vi "test-faketoggle.vi"() -> ()   [LabVIEW 2016]
uses:
  C:/Users/sciollalab/Documents/Brandeis-BNL/LabVIEW_Codes/BNL_ThermomechanicalStave/AerotechLibraries/Bin/Aerotech.A3200.dll
  AerotechLibraries/Bin/Aerotech.A3200.dll
panel:
  in  "error in (no error)":errorcluster
  in  "Axis Speeds":T1={"X [mm/s]"=10.0, "Y [mm/s]"=10.0, "Z [mm/s]"=10.0}
  out "Moving":bool
  in  "Program Errors":errorcluster
  out "XYZ Stage Control":refnum<k24>
  out "Stave origin":T2
  in  "XYZ Stage Frame: Coordinates for calibration":T3={"Stave origin"={"X [mm]"=-706.0, "Y [mm]"=140.5, "Z [mm]"=-13.5}, "Autofocus"={"X [mm]"=-686.0, "Y [mm]"=130.0, "Z [mm]"=-18.0}, "Calib Pattern"={"X [mm]"=-566.0, "Y [mm]"=39.26, "Z [mm]"=-22.0}}
  out "Current stage position [mm]":cluster{"X":dbl, "Y":dbl, "Z":dbl}
  in  "Update jog increment":bool
  in  "Jog step size":T2={"X [mm]"=0.1, "Y [mm]"=0.1, "Z [mm]"=0.1}
  in  "Backward":bool
  in  "Reset position":bool
  in  "Left":bool
  in  "Right":bool
  in  "Confirm position":bool
  in  "Forward":bool
  out "element":string
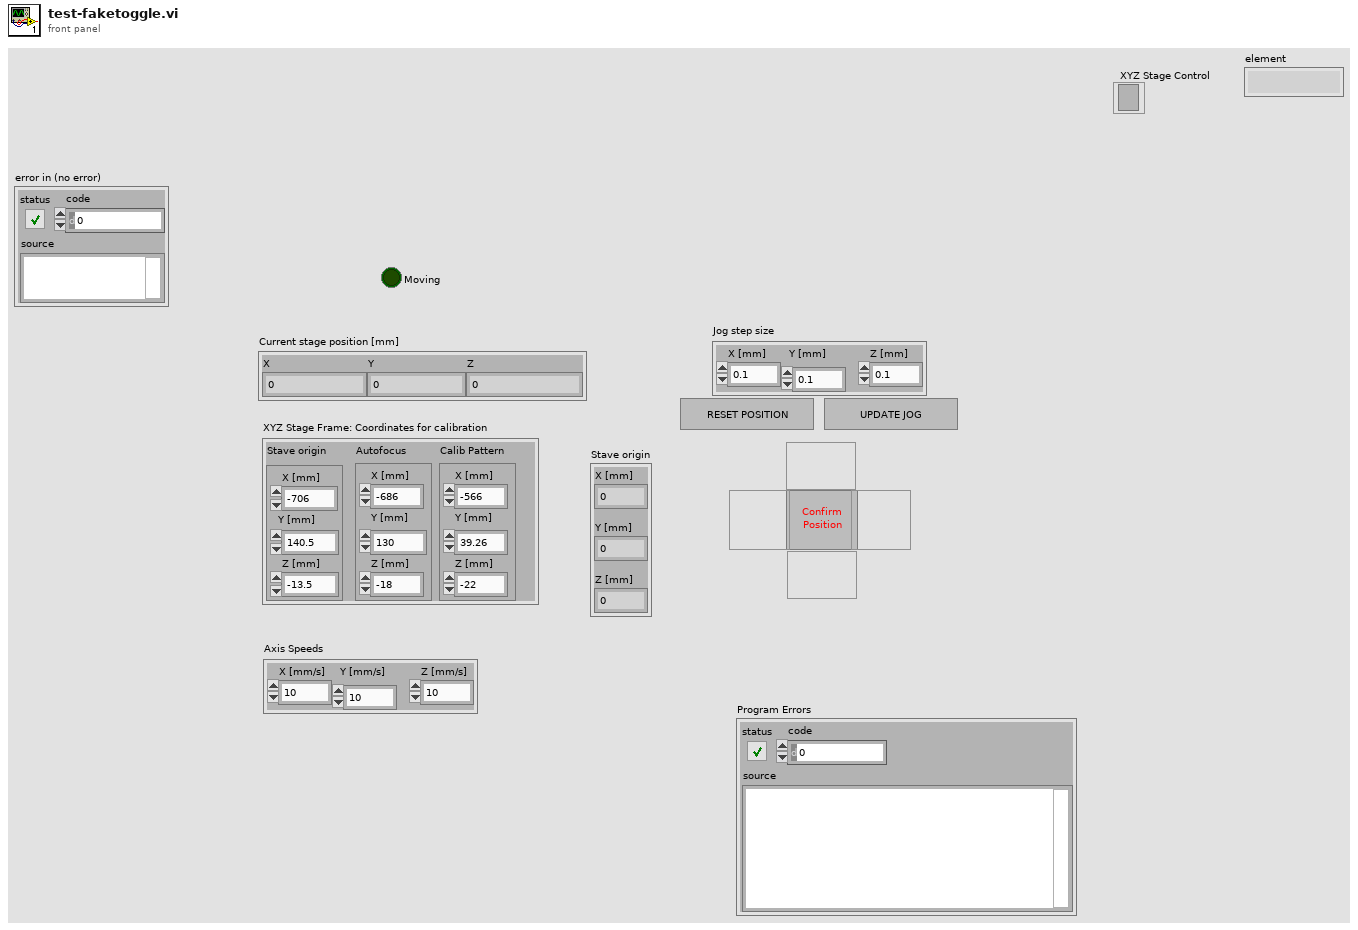
[diagram p1: front panel]
types:
  T1 = cluster{"X [mm/s]":dbl, "Y [mm/s]":dbl, "Z [mm/s]":dbl}
  T2 = cluster{"X [mm]":dbl, "Y [mm]":dbl, "Z [mm]":dbl}
  T3 = cluster{"Stave origin":cluster{"X [mm]":dbl, "Y [mm]":dbl, "Z [mm]":dbl}, "Autofocus":cluster{"X [mm]":dbl, "Y [mm]":dbl, "Z [mm]":dbl}, "Calib Pattern":cluster{"X [mm]":dbl, "Y [mm]":dbl, "Z [mm]":dbl}}
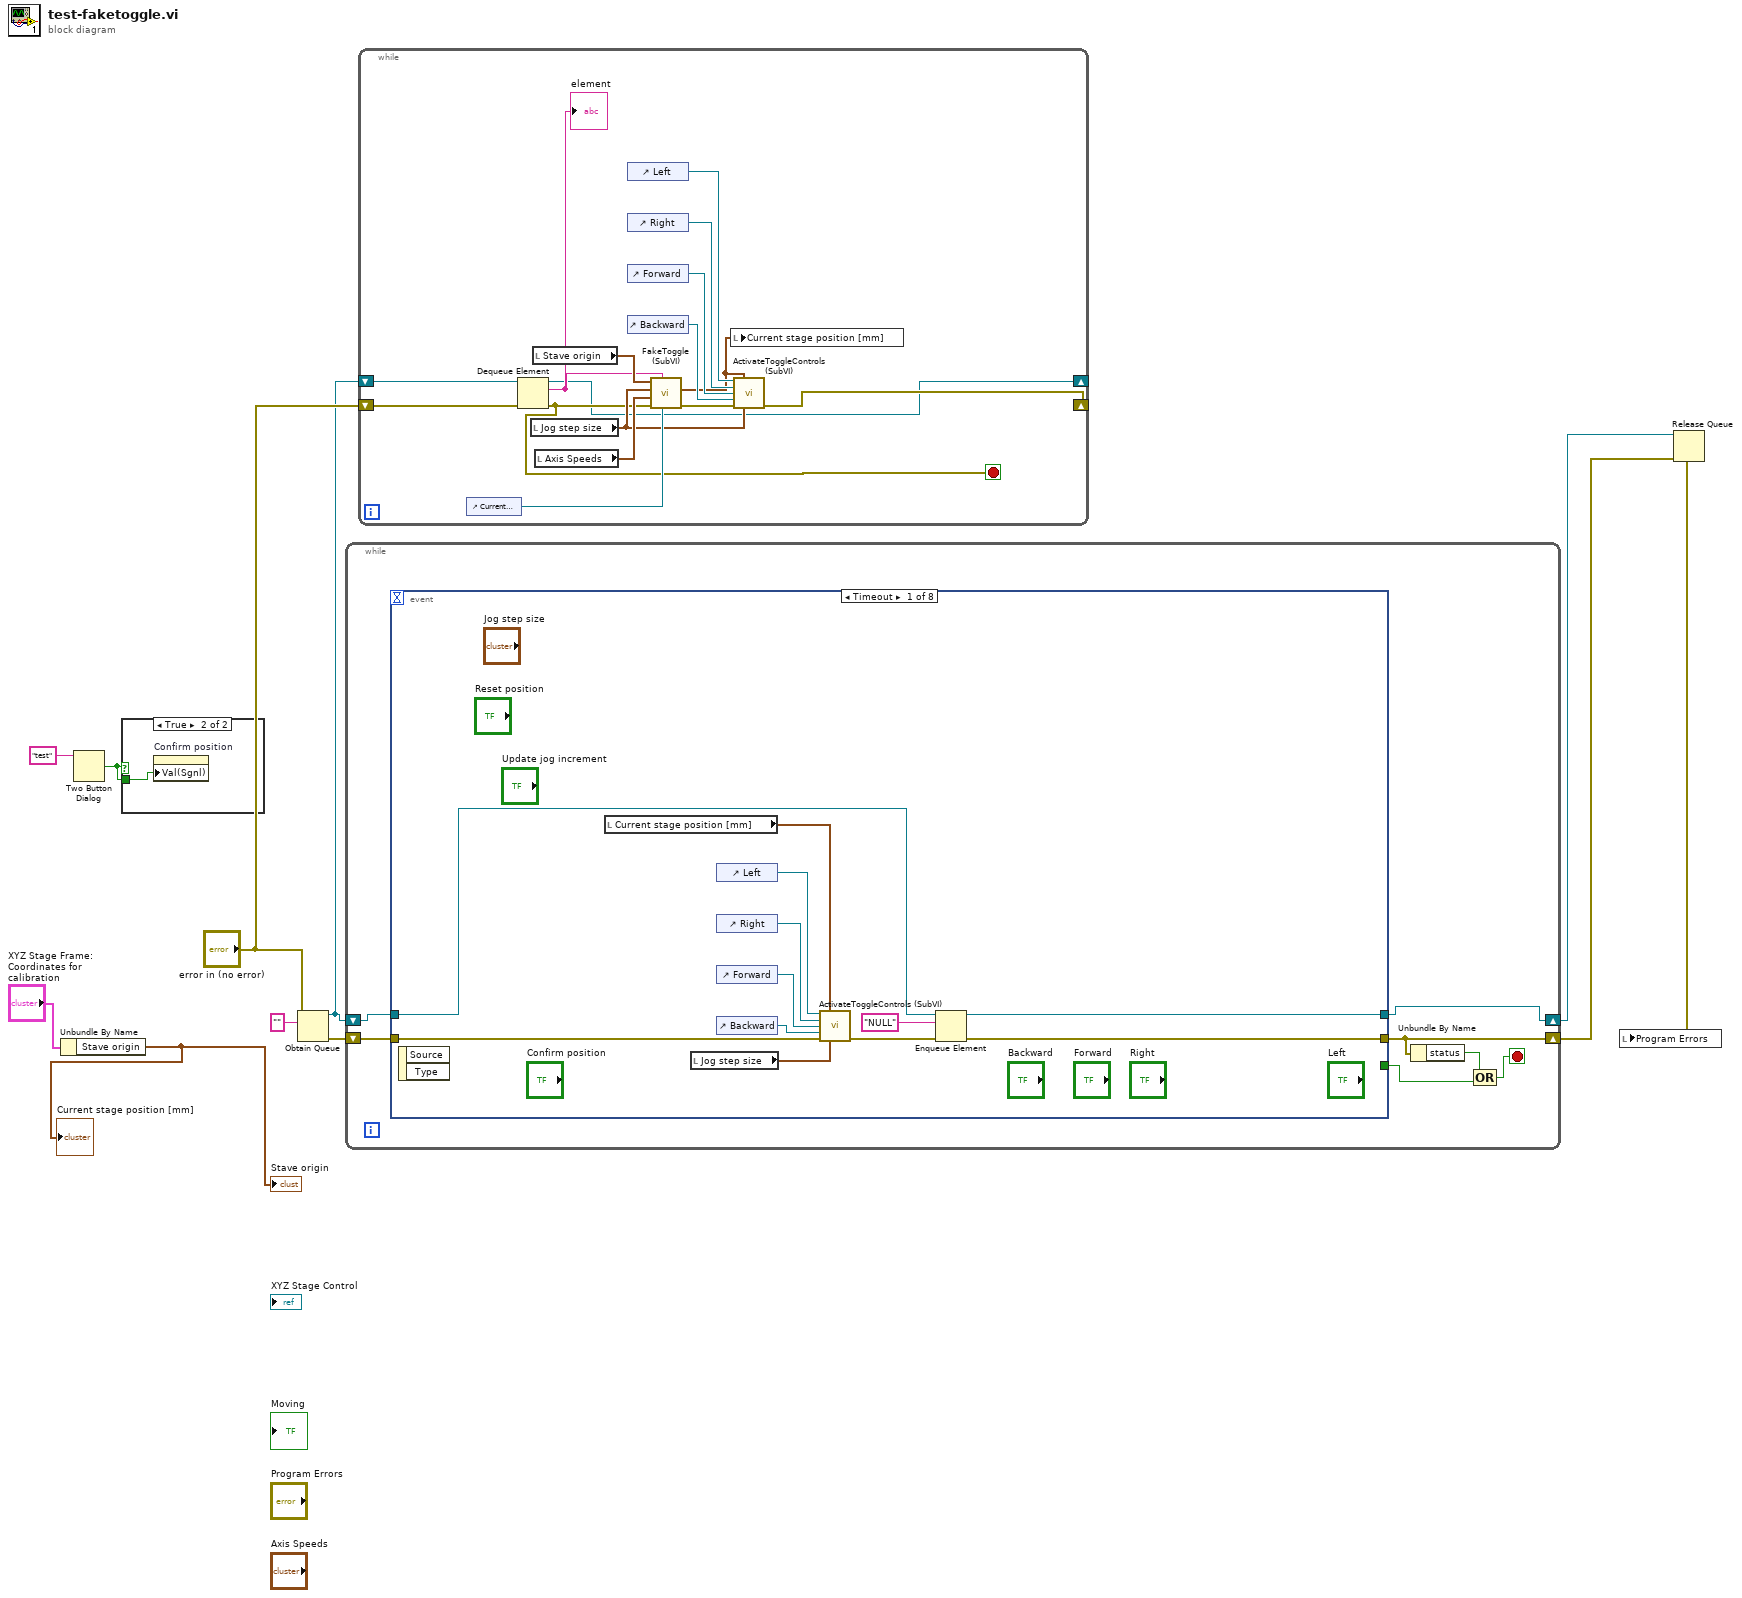
[diagram p0: block diagram]
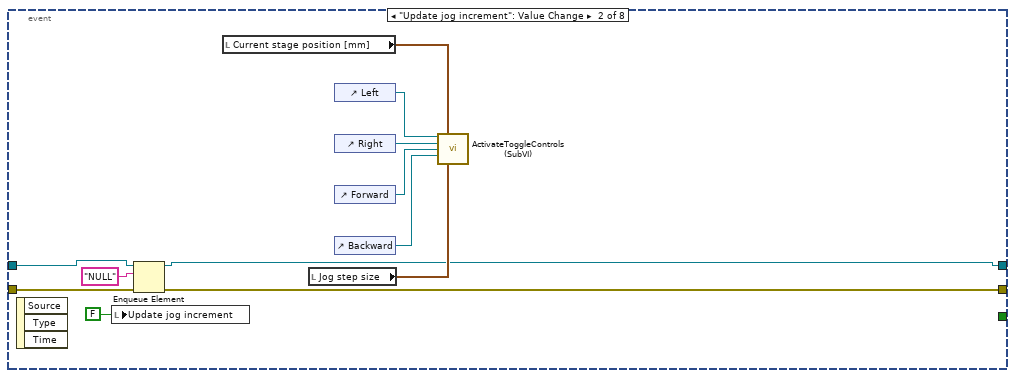
[diagram p3: hidden frame]
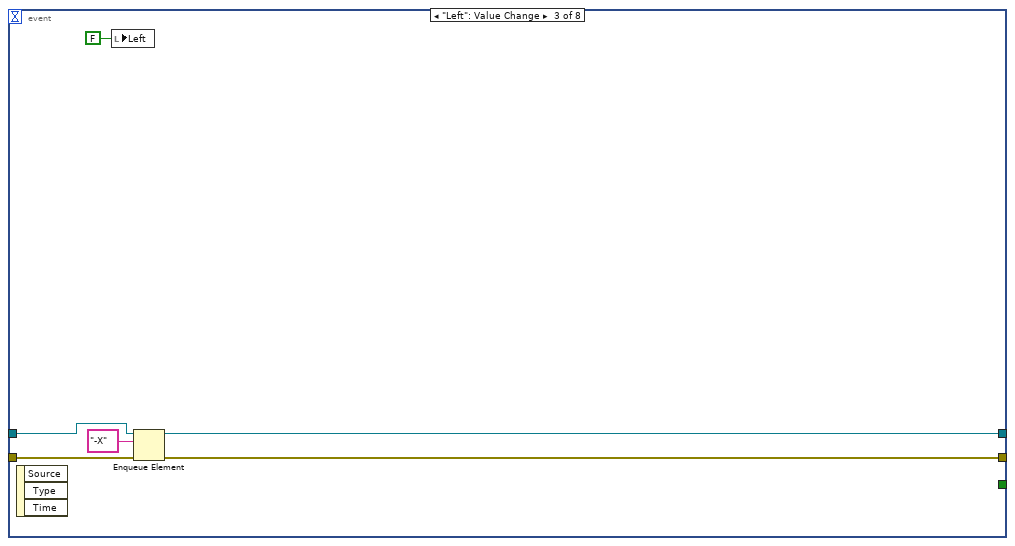
[diagram p4: hidden frame]
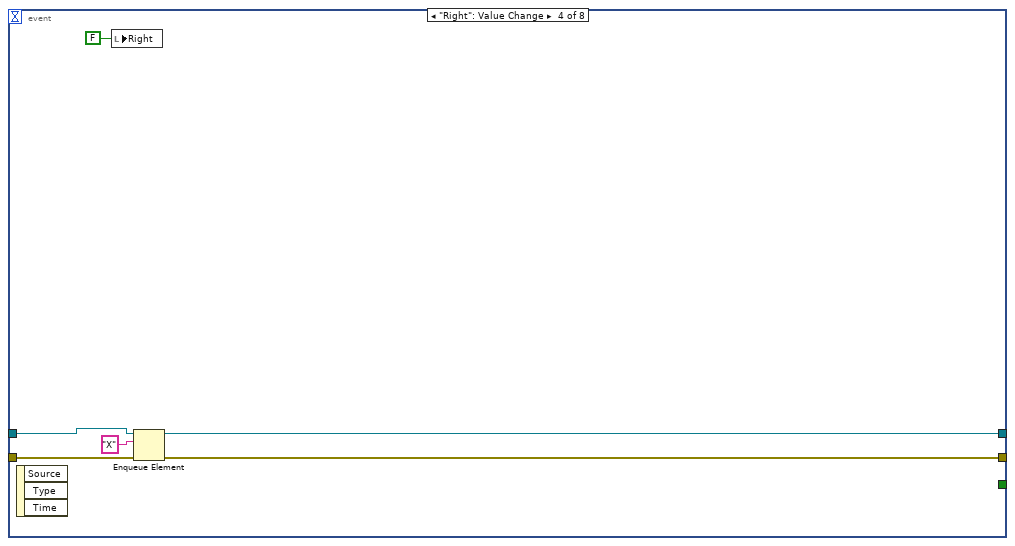
[diagram p5: hidden frame]
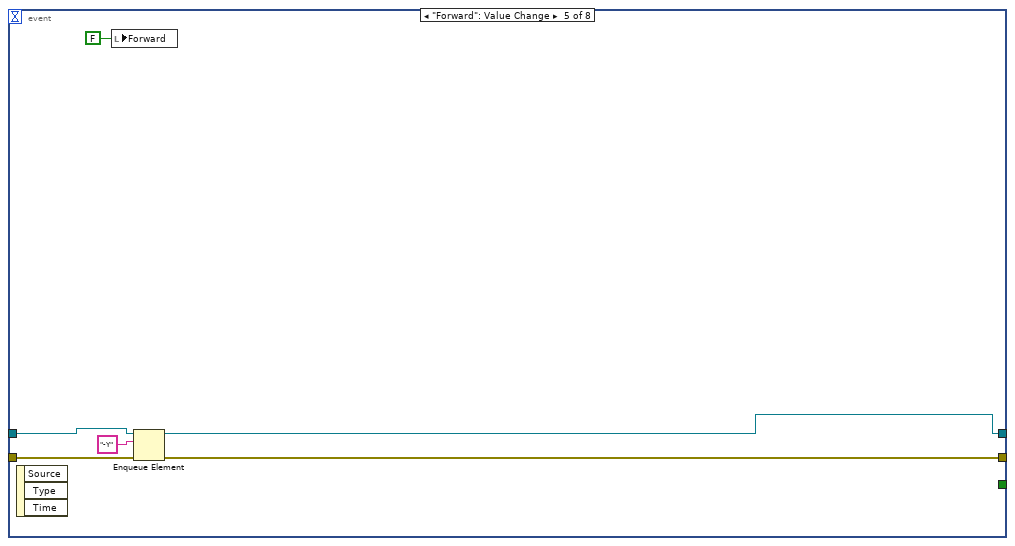
[diagram p6: hidden frame]
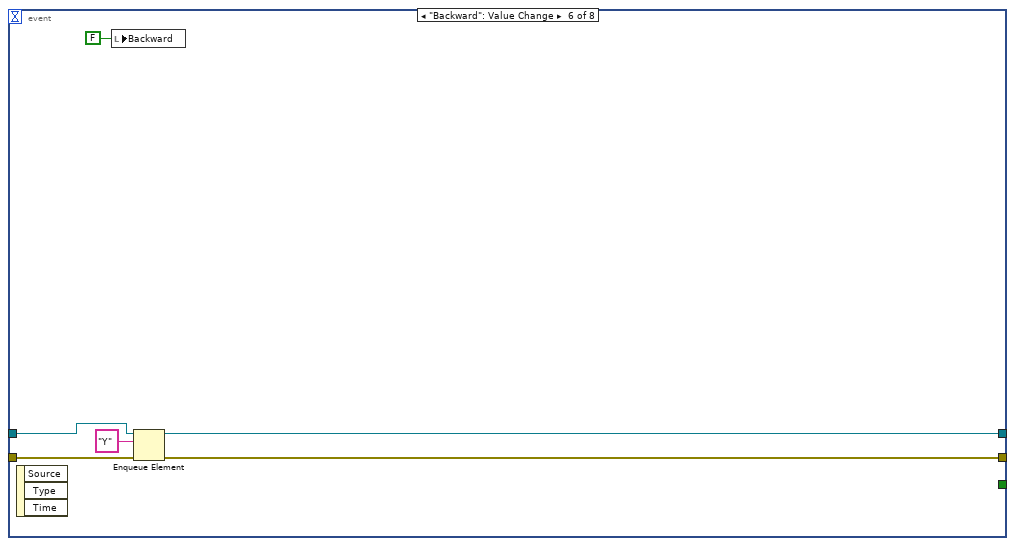
[diagram p7: hidden frame]
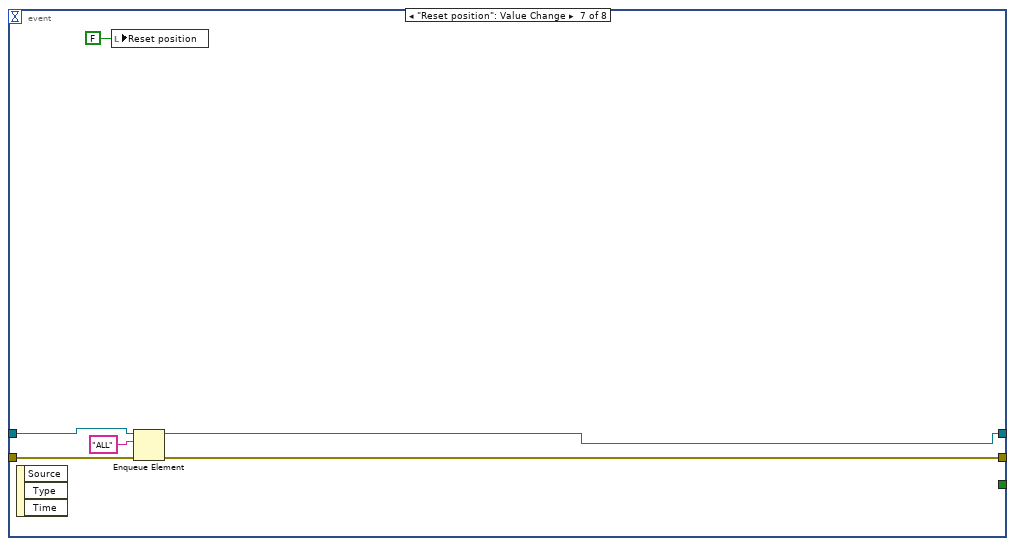
[diagram p8: hidden frame]
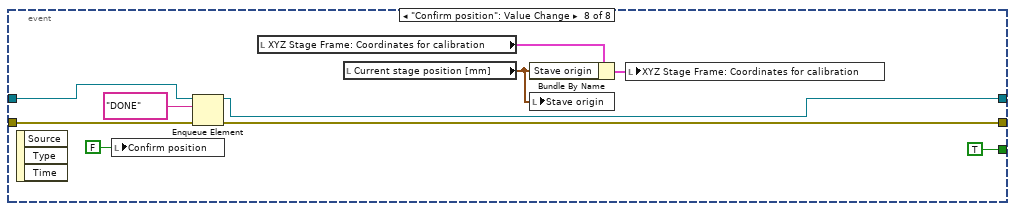
[diagram p9: hidden frame]
diagram:
  n1 = Unbundle By Name("XYZ Stage Frame: Coordinates for calibration") -> ("Stave origin"=→"Current stage position [mm]" →"Stave origin":T2)
  n2 = Two Button Dialog(message="test") -> (T button?=w1:bool)  [unwired: 2 in]
  n3 = case shown="True" w1 {
    tunnel: w1 -> [_ w12]
    frame False {
    }
    frame True {
      n4 = property on="Confirm position" class="Bool (strict)"("Val(Sgnl)"=w12) -> ()  [unwired: 2 in, 2 out]
    }
  }
  n5 = Obtain Queue(element data type="", error in (no error)="error in (no error)") -> (queue out=w5:refnum<queue>, error out=w11:errorcluster)  [unwired: 3 in, 1 out]
  n6 = while {
    shift-right: [w18] -> w3
    shift-left: w11 -> [w19]
    shift-right: [w13] -> w4
    shift-left: w5 -> [w14]
    stop <- w16 stop-if-true
    n7 = event shown="[0] Timeout" {
      selector: _ -> [_ _ _ _ _ _ _ _]
      dyn-events: _ -> [_ _ _ _ _ _ _ _]
      timeout: _ -> [_ _ _ _ _ _ _ _]
      tunnel: w14 -> [w24 w35 w47 w52 w60 w65 w72 w78]
      tunnel: w19 -> [w21 w34 w46 w54 w58 w64 w70 w75]
      tunnel: [w23 w33 w45 w53 w57 w63 w69 w76] -> w18
      tunnel: [_ _ _ _ _ _ _ TRUE] -> w15
      tunnel: [w20 w32 w44 w50 w56 w62 w68 w74] -> w13
      event Timeout {
        n8 = event-data() -> ()  [unwired: 1 in, 2 out]
        n9 = local read "Current stage position [mm]"() -> (w30:cluster{"X":dbl, "Y":dbl, "Z":dbl})
        n10 = local read "Jog step size"() -> (w31:T2)
        n11 = control-ref of="Left"() -> (w26:refnum<vi>)
        n12 = control-ref of="Right"() -> (w27:refnum<vi>)
        n13 = control-ref of="Forward"() -> (w28:refnum<vi>)
        n14 = control-ref of="Backward"() -> (w29:refnum<vi>)
        n15 = call "ActivateToggleControls (SubVI).vi"("Left refnum"=w26, "Current stage position [mm]"=w30, "Right refnum"=w27, "Forward refnum"=w28, "Backward refnum"=w29, "error in (no error)"=w21, "Jog step size"=w31) -> ("error out"=w22:errorcluster)  [unwired: 8 in]
        n16 = Enqueue Element(queue=w24, element="NULL", error in (no error)=w22) -> (queue out=w20:refnum<queue>, error out=w23:errorcluster)  [unwired: 1 in, 1 out]
      }
      event "Update jog increment": Value Change {
        n17 = event-data() -> ()  [unwired: 1 in, 3 out]
        n18 = local write "Update jog increment"(FALSE ("Update jog increment")) -> ()
        n19 = Enqueue Element(queue=w35, element="NULL", error in (no error)=w34) -> (queue out=w32:refnum<queue>, error out=w33:errorcluster)  [unwired: 1 in, 1 out]
        n20 = local read "Current stage position [mm]"() -> (w38:cluster{"X":dbl, "Y":dbl, "Z":dbl})
        n21 = local read "Jog step size"() -> (w39:T2)
        n22 = control-ref of="Left"() -> (w40:refnum<vi>)
        n23 = control-ref of="Right"() -> (w41:refnum<vi>)
        n24 = control-ref of="Forward"() -> (w42:refnum<vi>)
        n25 = control-ref of="Backward"() -> (w43:refnum<vi>)
        n26 = call "ActivateToggleControls (SubVI).vi"("Left refnum"=w40, "Current stage position [mm]"=w38, "Right refnum"=w41, "Forward refnum"=w42, "Backward refnum"=w43, "Jog step size"=w39) -> ()  [unwired: 9 in, 1 out]
      }
      event "Left": Value Change {
        n27 = event-data() -> ()  [unwired: 1 in, 3 out]
        n28 = local write "Left"(FALSE ("Left")) -> ()
        n29 = Enqueue Element(queue=w47, element="-X", error in (no error)=w46) -> (queue out=w44:refnum<queue>, error out=w45:errorcluster)  [unwired: 1 in, 1 out]
      }
      event "Right": Value Change {
        n30 = event-data() -> ()  [unwired: 1 in, 3 out]
        n31 = local write "Right"(FALSE ("Left")) -> ()
        n32 = Enqueue Element(queue=w52, element="X", error in (no error)=w54) -> (queue out=w50:refnum<queue>, error out=w53:errorcluster)  [unwired: 1 in, 1 out]
      }
      event "Forward": Value Change {
        n33 = event-data() -> ()  [unwired: 1 in, 3 out]
        n34 = local write "Forward"(FALSE ("Left")) -> ()
        n35 = Enqueue Element(queue=w60, element="-Y", error in (no error)=w58) -> (queue out=w56:refnum<queue>, error out=w57:errorcluster)  [unwired: 1 in, 1 out]
      }
      event "Backward": Value Change {
        n36 = event-data() -> ()  [unwired: 1 in, 3 out]
        n37 = local write "Backward"(FALSE ("Left")) -> ()
        n38 = Enqueue Element(queue=w65, element="Y", error in (no error)=w64) -> (queue out=w62:refnum<queue>, error out=w63:errorcluster)  [unwired: 1 in, 1 out]
      }
      event "Reset position": Value Change {
        n39 = event-data() -> ()  [unwired: 1 in, 3 out]
        n40 = local write "Reset position"(FALSE ("Reset position")) -> ()
        n41 = Enqueue Element(queue=w72, element="ALL", error in (no error)=w70) -> (queue out=w68:refnum<queue>, error out=w69:errorcluster)  [unwired: 1 in, 1 out]
      }
      event "Confirm position": Value Change {
        n42 = event-data() -> ()  [unwired: 1 in, 3 out]
        n43 = local write "Confirm position"(FALSE ("Confirm position")) -> ()
        n44 = Enqueue Element(queue=w78, element="DONE", error in (no error)=w75) -> (queue out=w74:refnum<queue>, error out=w76:errorcluster)  [unwired: 1 in, 1 out]
        n45 = local read "XYZ Stage Frame: Coordinates for calibration"() -> (w81:T3)
        n46 = local read "Current stage position [mm]"() -> (w80:cluster{"X":dbl, "Y":dbl, "Z":dbl})
        n47 = Bundle By Name(cluster=w81, "Stave origin"=w80) -> (w82:T3)
        n48 = local write "Stave origin"(w80) -> ()
        n49 = local write "XYZ Stage Frame: Coordinates for calibration"(w82) -> ()
      }
    }
    n50 = Unbundle By Name(w18) -> ("status"=w17:bool)
    n51 = Compound Arithmetic op=OR(w17, w15) -> (w16:bool)
  }
  n52 = while {
    shift-right: [w85] -> _
    shift-left: "error in (no error)" -> [w87]
    shift-right: [w84] -> _
    shift-left: w5 -> [w99]
    stop <- w86 stop-if-true
    n53 = control-ref of="Current stage position [mm]"() -> (w96:refnum<vi>)
    n54 = Dequeue Element(queue=w99, error in (no error)=w87) -> (queue out=w84:refnum<queue>, element=w95:string, error out=w86:errorcluster)  [unwired: 1 in, 1 out]
    "element" <- w95
    n55 = local read "Jog step size"() -> (w89:T2)
    n56 = local read "Stave origin"() -> (w98:T2)
    n57 = local read "Axis Speeds"() -> (w97:T1)
    n58 = control-ref of="Left"() -> (w94:refnum<vi>)
    n59 = control-ref of="Right"() -> (w93:refnum<vi>)
    n60 = control-ref of="Forward"() -> (w92:refnum<vi>)
    n61 = control-ref of="Backward"() -> (w91:refnum<vi>)
    n62 = call "FakeToggle (SubVI).vi"("Stage position"=w96, "Motion direction"=w95, "error in (no error)"=w86, "Axis Speeds"=w97, "Jog step size"=w89, "Original position"=w98) -> ("error out"=w90:errorcluster, "Current stage position [mm]"=w88:cluster{"X":dbl, "Y":dbl, "Z":dbl})  [unwired: 4 in]
    n63 = local write "Current stage position [mm]"(w88) -> ()
    n64 = call "ActivateToggleControls (SubVI).vi"("Left refnum"=w94, "Current stage position [mm]"=w88, "Right refnum"=w93, "Forward refnum"=w92, "Backward refnum"=w91, "error in (no error)"=w90, "Jog step size"=w89) -> ("error out"=w85:errorcluster)  [unwired: 8 in]
  }
  n65 = Release Queue(queue=w4, error in (no error)=w3) -> (error out=w9:errorcluster)  [unwired: 1 in, 2 out]
  n66 = local write "Program Errors"(w9) -> ()
